vi "Read AVI File.vi"() -> ()   [LabVIEW 2021]
doc: "This example shows how to open, read, and display an AVI file in NI Vision. The VI reads the frames per second property and plays the images back at the rate specified by the AVI file."
uses:
  QMH/Framework_lib.lvlib
panel:
  out "Number of Frames":u32
  out "Image_output":T1(plugin-control)
  in  "FPS":dbl(slide) scale=0.0..100.0
  out "init Frames Per Second":u32
  out "interframe latency":u32(graph)
  out "Progress Bar":i32(slide) max=9000 scale=1.0..9000.0
  in  "Stop":bool
  out "Image":T1(plugin-control)
  # "Overview: Demonstrate the use of the AVI functions to read an AVI movie file.\nRequirements: Vision Development Software.\nInstructions: Run the VI."
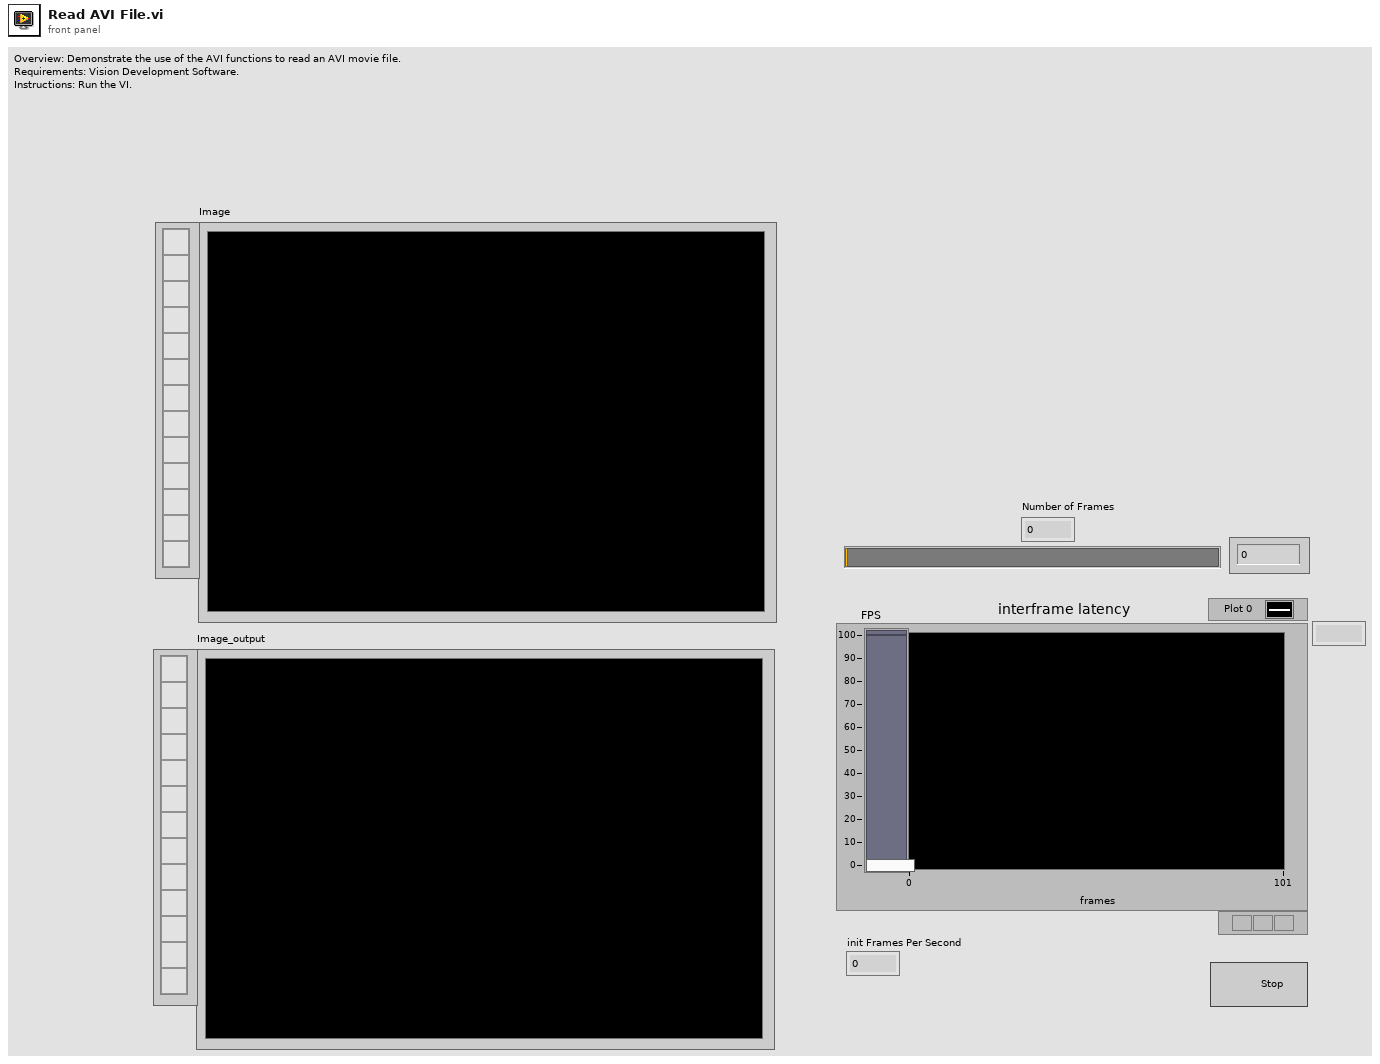
[diagram p1: front panel]
types:
  T1 = typedef "IMAQ Image.ctl" = refnum<image>
  T2 = typedef "IMAQ AVI2 Refnum.ctl" = refnum<k20>
  T3 = typedef "Image Type" = u32
  T4 = cluster{"Width":u32, "Height":u32, "Frames Per Second":u32, "Codec":string, "Has Data":bool}
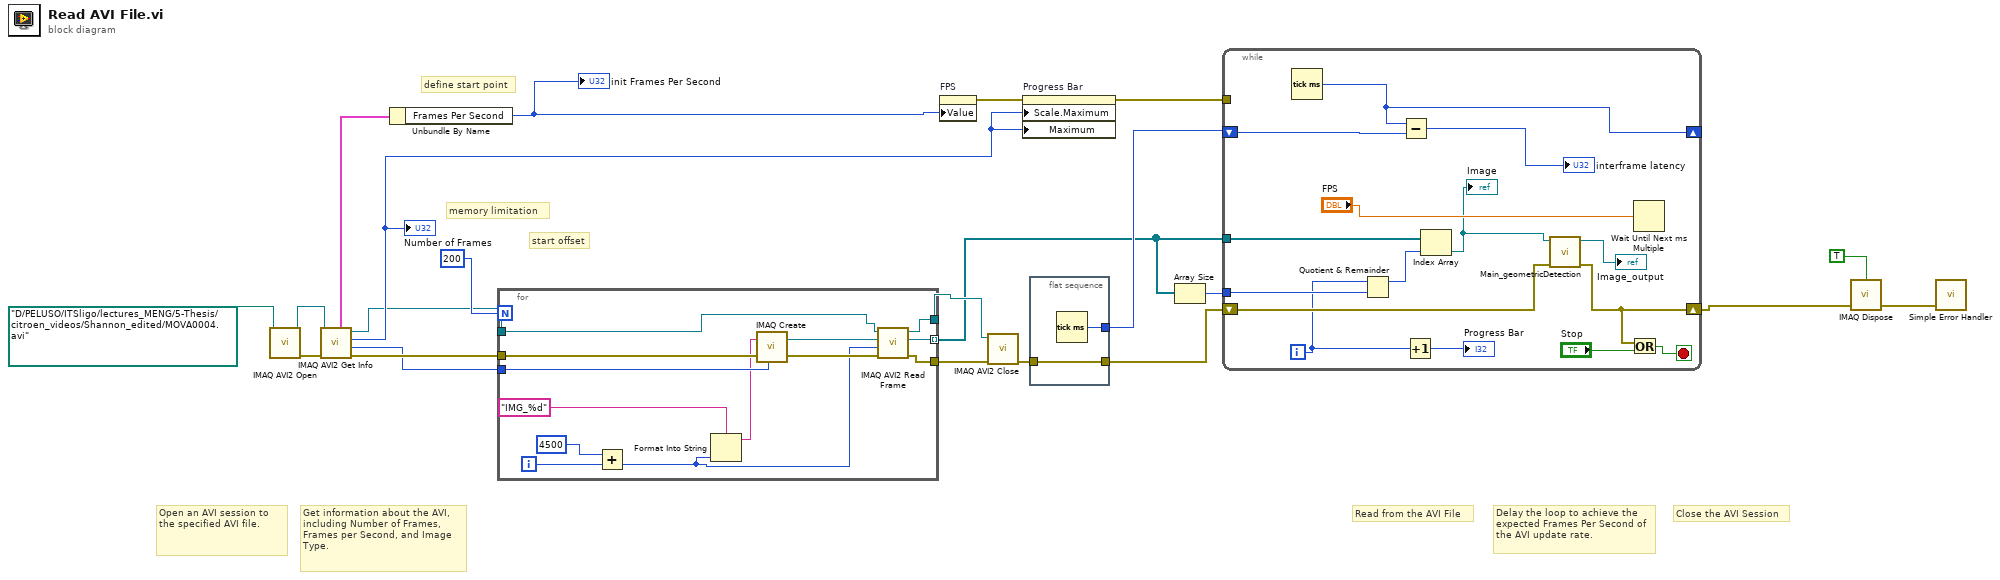
[diagram p0: block diagram]
diagram:
  # "start offset"
  # "memory limitation"
  # "define start point"
  # "Close the AVI Session"
  # "Read from the AVI File"
  # "Get information about the AVI, including Number of Frames, Frames per Second, and Image Type."
  # "Open an AVI session to the specified AVI file."
  # "Delay the loop to achieve the expected Frames Per Second of the AVI update rate."
  n1 = call "IMAQ AVI2 Open"("AVI File Path"=path "D:/PELUSO/ITSligo/lectures_MENG/5-Thesis/citroen_videos/Shannon_edited/MOVA0004.avi") -> ("error out"=w20:errorcluster, "AVI Refnum"=w19:T2)  [unwired: 2 in, 7 out]
  n2 = call "IMAQ AVI2 Get Info"("error in (no error)"=w20, "AVI Refnum"=w19) -> ("error out"=w18:errorcluster, "Image Type"=w16:T3, "Number of Frames"=w15:u32, "AVI Refnum (duplicate)"=w11:T2, "Frame Data"=w21:T4)  [unwired: 5 out]
  "Number of Frames" <- w15
  n3 = Unbundle By Name(w21) -> ("Frames Per Second"=w1:u32)
  "init Frames Per Second" <- w1
  n4 = for {
    N: 200 -> [_]
    tunnel: w18 -> [w35]
    tunnel: w16 -> [w34]
    tunnel: w11 -> [w28]
    tunnel: [w27] -> w4 mode=indexing
    tunnel: [w26] -> w10
    tunnel: [w25] -> w9
    i -> [w31]
    n5 = Add(x=4500, y=w31) -> (x+y=w24:i32)
    n6 = Format Into String(format string="IMG_%d", w24) -> (resulting string=w29:string)  [unwired: 2 in, 1 out]
    n7 = call "IMAQ Create"("Image Name"=w29, "Image Type"=w34, "error in (no error)"=w35) -> ("New Image"=w32:T1, "error out"=w33:errorcluster)  [unwired: 1 in, 1 out]
    n8 = call "IMAQ AVI2 Read Frame"("error in (no error)"=w33, "Frame Number"=w24, "Image"=w32, "AVI Refnum"=w28) -> ("error out"=w26:errorcluster, "Image Out"=w27:T1, "AVI Refnum (duplicate)"=w25:T2)  [unwired: 5 out]
  }
  n9 = property on="FPS" class="Slide (strict)"("Value"=w1) -> (error out=w2:errorcluster)  [unwired: 2 in, 1 out]
  n10 = call "IMAQ AVI2 Close"("error in (no error)"=w10, "AVI Refnum"=w9) -> ("error out"=w7:errorcluster)  [unwired: 9 out]
  n11 = property on="Progress Bar" class="Slide (strict)"(error in=w2, "Scale.Maximum"=w15, "Maximum"=w15) -> (error out=w14:errorcluster)  [unwired: 1 in, 1 out]
  n12 = flat-sequence {
    tunnel: w7 -> [w37]
    tunnel: [w37] -> w6
    tunnel: [w36] -> w5
    frame #0 {
      n13 = Tick Count (ms)() -> (millisecond timer value=w36:u32)
    }
  }
  n14 = Array Size(array=w4) -> (size(s)=w3:i32)
  n15 = while {
    tunnel: w14 -> [_]
    tunnel: w4 -> [w50]
    shift-right: [w41] -> w17
    shift-left: w6 -> [w42]
    shift-right: [w46] -> _
    shift-left: w5 -> [w48]
    tunnel: w3 -> [w44]
    i -> [w38]
    stop <- w49 stop-if-true
    n16 = Tick Count (ms)() -> (millisecond timer value=w46:u32)
    n17 = Quotient & Remainder(x=w38, y=w44) -> (x-y*floor(x/y)=w45:i32)  [unwired: 1 out]
    n18 = Subtract(x=w46, y=w48) -> (x-y=→"interframe latency":u32)
    n19 = Increment(x=w38) -> (x+1=→"Progress Bar":i32)
    n20 = Index Array(array=w50, index=w45) -> (element=w40:T1)
    "Image" <- w40
    n21 = call "Main_geometricDetection.vi"("error in (no error)"=w42, "input(RGB_U32)"=w40) -> ("error out"=w41:errorcluster, "output"=→"Image_output":T1)  [unwired: 8 in]
    n22 = Or(x=w41, y="Stop") -> (x .or. y?=w49:bool)
    n23 = Wait Until Next ms Multiple(millisecond multiple="FPS") -> ()  [unwired: 1 out]
  }
  n24 = call "IMAQ Dispose"("All Images? (No)"=TRUE, "error in (no error)"=w17) -> ("error out"=w22:errorcluster)  [unwired: 1 in, 3 out]
  n25 = call <vilib>:"Simple Error Handler.vi"("error in (no error)"=w22) -> ()  [unwired: 1 in, 8 out]
